vi "Servo Motors Control.vi"   [LabVIEW 2014]
doc: "This example shows how to control 180 deg servo motor using servo library. there are two method demostrated on this example,1.using degrees value for example 45 deg or 90 deg. 2. using pulse with (us)."
uses:
  QwaveSys_Interface/QwaveSys_Interface.lvlib
panel:
  # "Overview: Demonstrates how to control two 180 degree servo motors using Servo Motor API.\nRequirements: LabVIEW Full Development System,Arduino Compatible Compiler for LabVIEW,Programmable Wireless Stamp (PWS) Library.\nInstructions:\n1. Wire a servo motor#1 as specified below where the data pin is wired to the specified Digital Pin (GPIO5) below.\n2. Wire a servo motor#2 as specified below where the data pin is wired to the specified Digital Pin (GPIO15) below.\n3. If this example has been loaded from the Arduino Compatible Compiler for LabVIEW, simply select Compile and Download.  Otherwise, open Tools>Arduino Compatible Compiler for LabVIEW in LabVIEW, then select File>Load VI, and select this VI and then Compile and Download.\n4. Observed the servo motor #1 and #2 , Both of them will be toggled between 0 - 180 degree with 1 s delay."
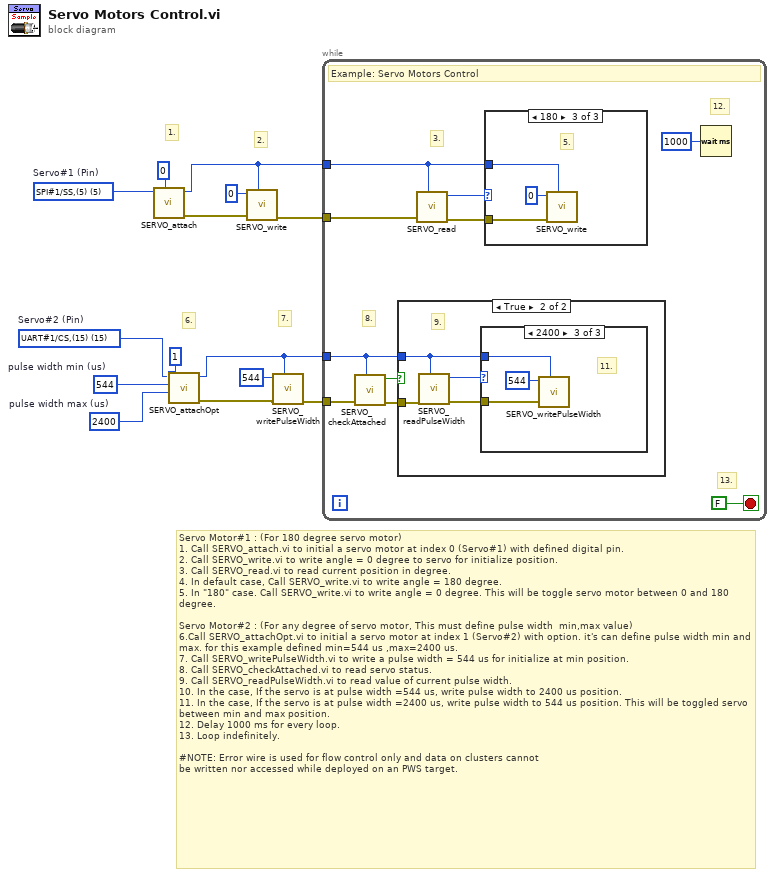
[diagram p0: block diagram]
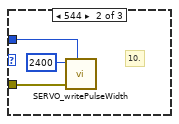
[diagram p4: hidden frame]
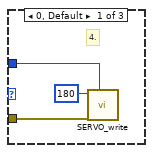
[diagram p5: hidden frame]
diagram:
  w1 = u8 15 items=["SPI#1/SS,(5)"=5, "SPI#2/MOSI,(13)"=13, "SPI#3/MISO,(12)"=12, "SPI#4/SCLK,(14)"=14, "UART#1/CS,(15)"=15, "UART#2/TXD,(1)"=1, "UART#3/RXD,(3)"=3, "UART#4/LED,(16)"=16, "FPROM_Btn,(0)"=0, "SDCard_CS,(4)"=4, "I2C-SDA/TXD1,(2)"=2, "ADC0,(17)"=17]  # Servo#2 (Pin)
  w2 = u8 5 items=["SPI#1/SS,(5)"=5, "SPI#2/MOSI,(13)"=13, "SPI#3/MISO,(12)"=12, "SPI#4/SCLK,(14)"=14, "UART#1/CS,(15)"=15, "UART#2/TXD,(1)"=1, "UART#3/RXD,(3)"=3, "UART#4/LED,(16)"=16, "FPROM_Btn,(0)"=0, "SDCard_CS,(4)"=4, "I2C-SDA/TXD1,(2)"=2, "ADC0,(17)"=17]  # Servo#1 (Pin)
  w4 = u16 2400  # pulse width max (us)
  w3 = u16 544  # pulse width min (us)
  # "Servo Motor#1 : (For 180 degree servo motor)\n1. Call SERVO_attach.vi to initial a servo motor at index 0 (Servo#1) with defined digital pin.\n2. Call SERVO_write.vi to write angle = 0 degree to servo for initialize position. \n3. Call SERVO_read.vi to read current position in degree.\n4. In default case, Call SERVO_write.vi to write angle = 180 degree.\n5. In \"180\" case. Call SERVO_write.vi to write angle = 0 degree. This will be toggle servo motor between 0 and 180 degree.\n\nServo Motor#2 : (For any degree of servo motor, This must define pulse width  min,max value)\n6.Call SERVO_attachOpt.vi to initial a servo motor at index 1 (Servo#2) with option. it's can define pulse width min and max. for this example defined min=544 us ,max=2400 us.\n7. Call SERVO_writePulseWidth.vi to write a pulse width = 544 us for initialize at min position. \n8. Call SERVO_checkAttached.vi to read servo status.\n9. Call SERVO_readPulseWidth.vi to read value of current pulse width.\n10. In the case, If the servo is at pulse width =544 us, write pulse width to 2400 us position.\n11. In the case, If the servo is at pulse width =2400 us, write pulse width to 544 us position. This will be toggled servo between min and max position.\n12. Delay 1000 ms for every loop.\n13. Loop indefinitely.\n\n#NOTE: Error wire is used for flow control only and data on clusters cannot\nbe written nor accessed while deployed on an PWS target."
  # "7."
  # "6."
  # "2."
  # "1."
  n1 = call "SERVO_attach.vi"("Interface (0-4)"=u8 0, "PIN"=w2) -> ("error out"=w13:errorcluster, "Instance"=w10:u8)  [unwired: 8 in]
  n2 = call "SERVO_attachOpt.vi"("Interface (0-4)"=u8 1, "pulse width max (us)"=w4, "pulse width min (us)"=w3, "PIN"=w1) -> ("error out"=w8:errorcluster, "Instance"=w6:u8)  [unwired: 6 in]
  n3 = call "SERVO_write.vi"("Instance"=w10, "error in (no error)"=w13, "angle"=u8 0) -> ("error out"=w11:errorcluster)  [unwired: 8 in]
  n4 = call "SERVO_writePulseWidth.vi"("Instance"=w6, "error in (no error)"=w8, "pulse width (us)"=u16 544) -> ("error out"=w9:errorcluster)  [unwired: 8 in]
  n5 = while {
    tunnel: w11 -> [w24]
    tunnel: w10 -> [w23]
    tunnel: w9 -> [w18]
    tunnel: w6 -> [w17]
    stop <- FALSE stop-if-true
    # "13."
    # "12."
    # "8."
    # "3."
    # "Example: Servo Motors Control"
    n6 = call "SERVO_checkAttached.vi"("Instance"=w17, "error in (no error)"=w18) -> ("error out"=w16:errorcluster, "attached"=w15:bool)  [unwired: 8 in]
    n7 = case shown="True" w15 {
      tunnel: w17 -> [_ w26]
      tunnel: w16 -> [_ w25]
      frame False {
      }
      frame True {
        # "9."
        n8 = call "SERVO_readPulseWidth.vi"("Instance"=w26, "error in (no error)"=w25) -> ("error out"=w28:errorcluster, "pulse width (us)"=w27:u16)  [unwired: 8 in]
        n9 = case shown="2400" w27 {
          tunnel: w28 -> [_ w31 w33]
          tunnel: w26 -> [_ w30 w32]
          frame 0, Default {
          }
          frame 544 {
            # "10."
            n10 = call "SERVO_writePulseWidth.vi"("Instance"=w30, "error in (no error)"=w31, "pulse width (us)"=u16 2400) -> ()  [unwired: 8 in, 1 out]
          }
          frame 2400 {
            # "11."
            n11 = call "SERVO_writePulseWidth.vi"("Instance"=w32, "error in (no error)"=w33, "pulse width (us)"=u16 544) -> ()  [unwired: 8 in, 1 out]
          }
        }
      }
    }
    n12 = call "SERVO_read.vi"("Instance"=w23, "error in (no error)"=w24) -> ("error out"=w20:errorcluster, "angle"=w21:u8)  [unwired: 8 in]
    n13 = case shown="180" w21 {
      tunnel: w20 -> [w37 _ w40]
      tunnel: w23 -> [w35 _ w38]
      frame 0, Default {
        # "4."
        n14 = call "SERVO_write.vi"("Instance"=w35, "error in (no error)"=w37, "angle"=u8 180) -> ()  [unwired: 8 in, 1 out]
      }
      frame 1..179 {
      }
      frame 180 {
        # "5."
        n15 = call "SERVO_write.vi"("Instance"=w38, "error in (no error)"=w40, "angle"=u8 0) -> ()  [unwired: 8 in, 1 out]
      }
    }
    n16 = Wait (ms)(milliseconds to wait=u32 1000) -> ()  [unwired: 1 out]
  }
